vi "Dummy Read Data.vi"(8 "error in (no error)":errorcluster, 11 "Actor in":refnum<class "Actor.lvclass">) -> (0 "error out":errorcluster, 2 "Boolean":bool, 3 "Actor out":refnum<class "Actor.lvclass">)   [LabVIEW 2014]
uses:
  <vilib>/ActorFramework/Actor/Actor.lvclass
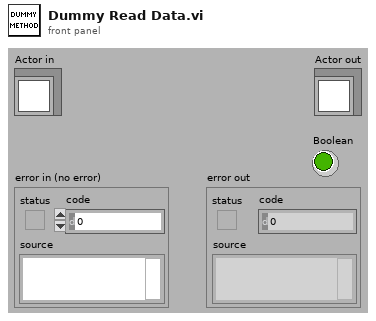
[diagram p1: front panel]
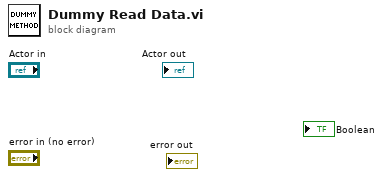
[diagram p0: block diagram]
diagram:
